vi "SRV_Sensor View Tab_DEMO.vi"() -> ()   [LabVIEW 2014]
uses:
  SRV_Sensor View Indicator Names.ctl
panel:
  in  "Close":bool
  out "Boolean 32":bool
  out "Boolean 31":bool
  out "Boolean 30":bool
  out "Boolean 29":bool
  out "Boolean 28":bool
  out "Boolean 27":bool
  out "Boolean 26":bool
  out "Boolean 25":bool
  out "Boolean 24":bool
  out "Boolean 23":bool
  out "Boolean 22":bool
  out "Boolean 21":bool
  out "Boolean 20":bool
  out "Boolean 19":bool
  out "Boolean 18":bool
  out "Boolean 17":bool
  out "Boolean 16":bool
  out "Boolean 15":bool
  out "Boolean 14":bool
  out "Boolean 13":bool
  out "Boolean 12":bool
  out "Boolean 11":bool
  out "Boolean 10":bool
  out "Boolean 9":bool
  out "Boolean 8":bool
  out "Boolean 7":bool
  out "Boolean 6":bool
  out "Boolean 5":bool
  out "Boolean 4":bool
  out "Boolean 3":bool
  out "Boolean 2":bool
  out "Boolean 01":bool
  out "Numeric 08":dbl
  out "Numeric 07":dbl
  out "Numeric 06":dbl
  out "Numeric 05":dbl
  out "Numeric 04":dbl
  out "Numeric 03":dbl
  out "Numeric 02":dbl
  out "Numeric 01":dbl
  out "Meter 04":dbl(knob) scale=0.0..10.0
  out "Meter 03":dbl(knob) scale=0.0..10.0
  out "Meter 02":dbl(knob) scale=0.0..10.0
  out "Meter 01":dbl(knob) scale=0.0..10.0
  out "Gauge 04":dbl(knob) scale=0.0..10.0
  out "Gauge 03":dbl(knob) scale=0.0..10.0
  out "Gauge 02":dbl(knob) scale=0.0..10.0
  out "Right Distance":dbl(knob) scale=0.0..100.0 scale format="%#.3g"
  in  "Sensor View Indicator Names":T1=enum."Gauge 01"
  # "Sensor View Tab"
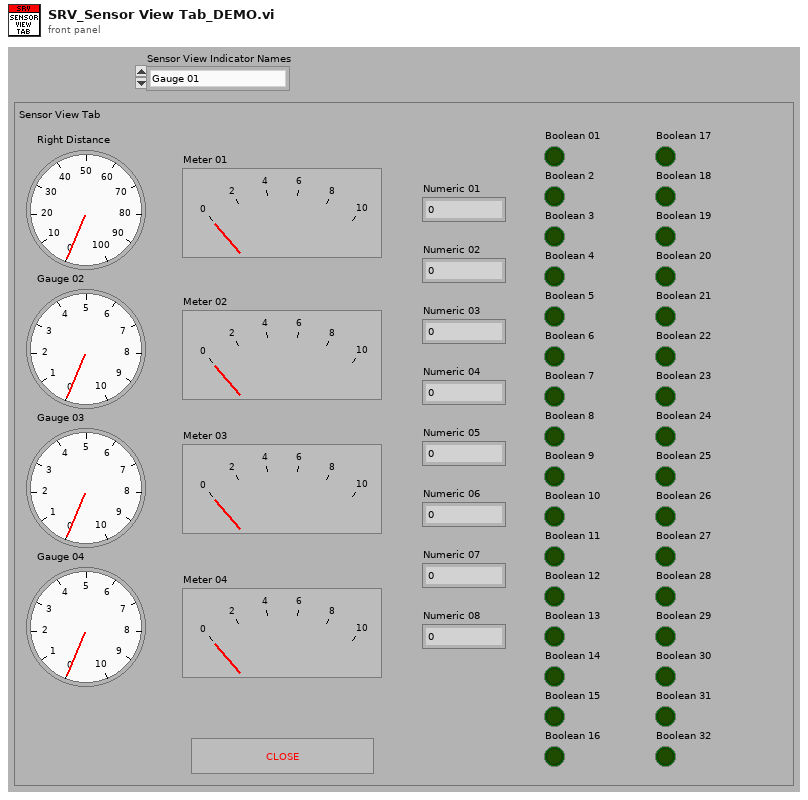
[diagram p1: front panel]
types:
  T1 = typedef "SRV_Sensor View Indicator Names.ctl" = enum16{"None", "Gauge 01", "Gauge 02", "Gauge 03", "Gauge 04", "Meter 01", "Meter 02", "Meter 03", "Meter 04", "Numeric 01", "Numeric 02", "Numeric 03", "Numeric 04", "Numeric 05", "Numeric 06", "Numeric 07", "Numeric 08", "Boolean 01", "Boolean 02", "Boolean 03", "Boolean 04", "Boolean 05", "Boolean 06", "Boolean 07", "Boolean 08", "Boolean 09", "Boolean 10", "Boolean 11", "Boolean 12", "Boolean 13", "Boolean 14", "Boolean 15", "Boolean 16", "Boolean 17", "Boolean 18", "Boolean 19", "Boolean 20", "Boolean 21", "Boolean 22", "Boolean 23", "Boolean 24", "Boolean 25", "Boolean 26", "Boolean 27", "Boolean 28", "Boolean 29", "Boolean 30", "Boolean 31", "Boolean 32"}
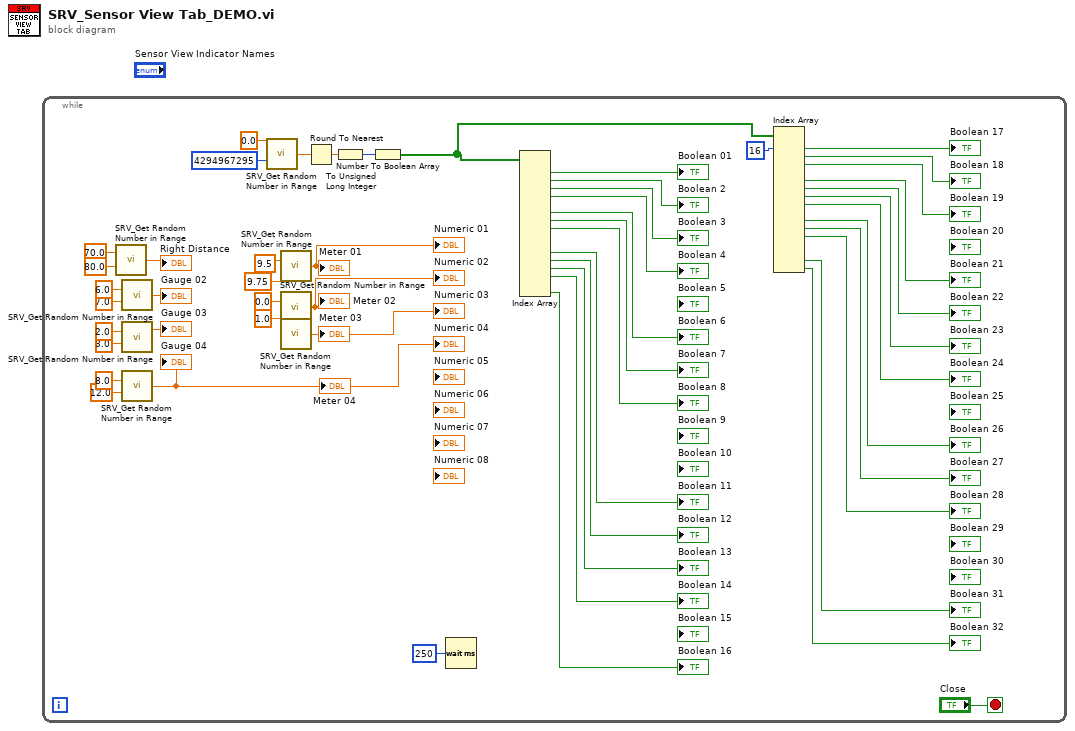
[diagram p0: block diagram]
diagram:
  n1 = while {
    stop <- "Close" stop-if-true
    n2 = call "SRV_Get Random Number in Range.vi"("Low (0)"=70.0 ("Low"), "High (10)"=80.0 ("High")) -> ("Random Number"=→"Right Distance":dbl)  [unwired: 13 in]
    n3 = call "SRV_Get Random Number in Range.vi"("Low (0)"=6.0, "High (10)"=7.0) -> ("Random Number"=→"Gauge 02":dbl)  [unwired: 13 in]
    n4 = call "SRV_Get Random Number in Range.vi"("Low (0)"=2.0, "High (10)"=3.0) -> ("Random Number"=→"Gauge 03":dbl)  [unwired: 13 in]
    n5 = call "SRV_Get Random Number in Range.vi"("Low (0)"=8.0, "High (10)"=12.0) -> ("Random Number"=→"Gauge 04" →"Meter 04" →"Numeric 04":dbl)  [unwired: 13 in]
    n6 = call "SRV_Get Random Number in Range.vi"("Low (0)"=0.0, "High (10)"=u32 4294967295) -> ("Random Number"=w29:dbl)  [unwired: 13 in]
    n7 = call "SRV_Get Random Number in Range.vi"("Low (0)"=9.5, "High (10)"=9.75) -> ("Random Number"=→"Meter 01" →"Numeric 01":dbl)  [unwired: 13 in]
    n8 = call "SRV_Get Random Number in Range.vi"("Low (0)"=0.0, "High (10)"=1.0) -> ("Random Number"=→"Meter 02" →"Numeric 02":dbl)  [unwired: 13 in]
    n9 = call "SRV_Get Random Number in Range.vi"() -> ("Random Number"=→"Meter 03" →"Numeric 03":dbl)  [unwired: 15 in]
    n10 = Round To Nearest(number=w29) -> (nearest integer value=w28:dbl)
    n11 = To Unsigned Long Integer(number=w28) -> (unsigned 32bit integer=w27:u32)
    n12 = Number To Boolean Array(number=w27) -> (Boolean array=w13:bool[])
    n13 = Wait (ms)(milliseconds to wait=u32 250) -> ()  [unwired: 1 out]
    n14 = Index Array(array=w13) -> (element #1=→"Boolean 01":bool, element #2=→"Boolean 2":bool, element #3=→"Boolean 3":bool, element #4=→"Boolean 4":bool, element #6=→"Boolean 6":bool, element #7=→"Boolean 7":bool, element #8=→"Boolean 8":bool, element #11=→"Boolean 11":bool, element #12=→"Boolean 12":bool, element #13=→"Boolean 13":bool, element #14=→"Boolean 14":bool, element #16=→"Boolean 16":bool)  [unwired: 16 in, 4 out]
    n15 = Index Array(array=w13, index #1=16 ("index")) -> (element #1=→"Boolean 17":bool, element #2=→"Boolean 18":bool, element #3=→"Boolean 19":bool, element #5=→"Boolean 21":bool, element #6=→"Boolean 22":bool, element #7=→"Boolean 23":bool, element #8=→"Boolean 24":bool, element #10=→"Boolean 26":bool, element #11=→"Boolean 27":bool, element #12=→"Boolean 28":bool, element #15=→"Boolean 31":bool, element #16=→"Boolean 32":bool)  [unwired: 15 in, 4 out]
  }
